vi "real-time-temperature-monitoring.vi"() -> ()   [LabVIEW 2025]
uses:
  <vilib>/numeric/sub_Random U32.vi
  <vilib>/numeric/Random Number (Range) U64.vi
panel:
  in  "Boolean":bool
  out "temp":dbl
  out "Waveform Chart":u64(graph)
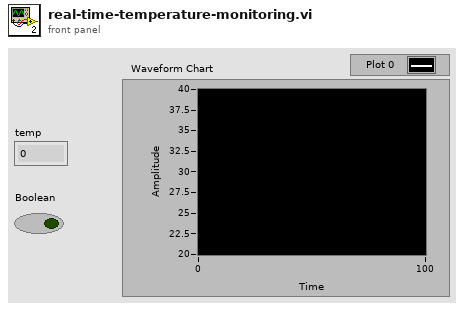
[diagram p1: front panel]
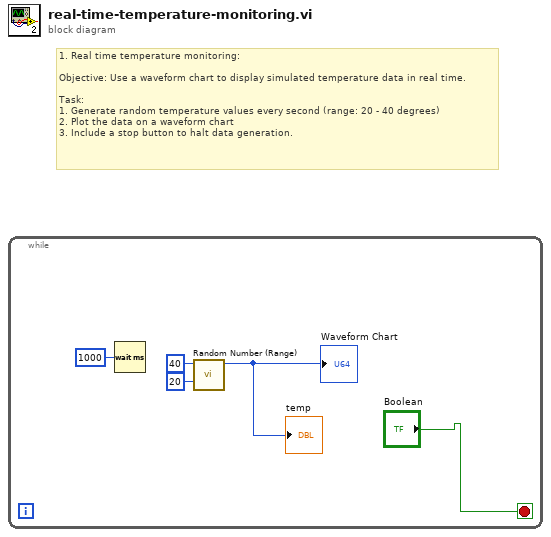
[diagram p0: block diagram]
diagram:
  # "1. Real time temperature monitoring:\n\nObjective: Use a waveform chart to display simulated temperature data in real time.\n\nTask:\n1. Generate random temperature values every second (range: 20 - 40 degrees)\n2. Plot the data on a waveform chart\n3. Include a stop button to halt data generation."
  n1 = while {
    stop <- "Boolean" stop-if-true
    n2 = Wait (ms)(milliseconds to wait=u32 1000) -> ()  [unwired: 1 out]
    n3 = call-poly <vilib>:"Random Number (Range).vi"("lower bound (0)"=u64 20, "upper bound (100)"=u64 40) -> ("number"=→"Waveform Chart" →"temp":u64)  [unwired: 9 in]
  }
